vi "GlyphFactory_Init.vi"(8 "error in (no error)":errorcluster, 11 "reference in":refnum<class "GlyphFactory.lvclass"> caption="This control should only be used when\na sub class is inheriting this class") -> (0 "error out":errorcluster, 3 "reference out":refnum<class "GlyphFactory.lvclass"> caption="This indicator should only be used when\na sub class is inheriting this class")   [LabVIEW 2012, in "GlyphFactory.lvclass"]
uses:
  GlyphFactory.lvclass
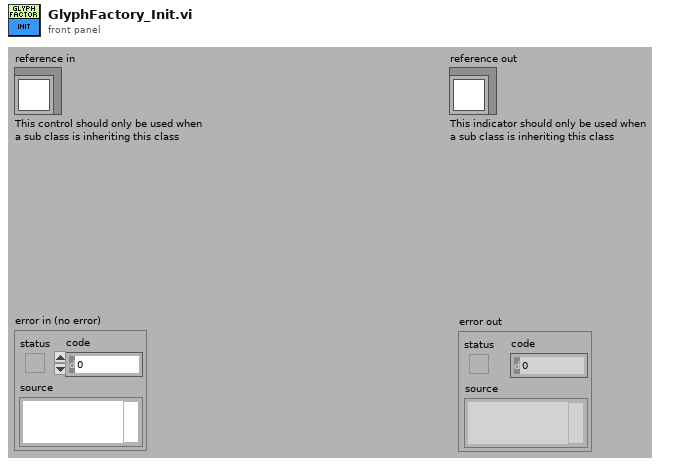
[diagram p1: front panel]
types:
  T1 = typedef "GlyphFactory.lvclass/ObjectAttributes.ctl" = cluster{"CharObjectTypes":cluster{"Char":string, "Text Color":u32, "Font":cluster{"Font Name:":string, "Size":i16, "Strikeout?":bool, "Italic?":bool, "Underline?":bool, "Outline?":bool, "Shadow?":bool, "Bold?":bool}}[], "CharObjects":refnum<class "Character.lvclass">[]}
  T2 = cluster{"Char":string, "Text Color":u32, "Font":cluster{"Font Name:":string, "Size":i16, "Strikeout?":bool, "Italic?":bool, "Underline?":bool, "Outline?":bool, "Shadow?":bool, "Bold?":bool}}[]
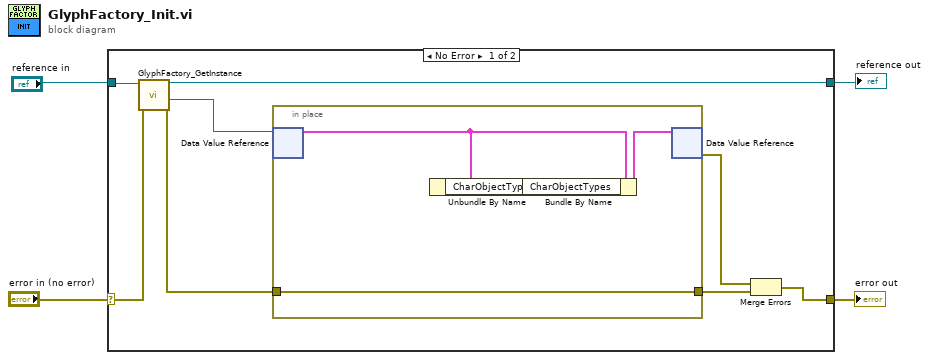
[diagram p0: block diagram]
diagram:
  n1 = case shown="No Error" "error in (no error)" {
    selector: "error in (no error)" -> [w10 w18]
    tunnel: [w11 w18] -> w3
    tunnel: "reference in" -> [w9 w17]
    tunnel: [w7 w17] -> w1
    frame No Error {
      n2 = call "GlyphFactory_GetInstance.vi"("error in (no error)"=w10, "reference in"=w9) -> ("error out"=w6:errorcluster, "DVRRefOut"=w8:refnum<data-value>, "reference out"=w7:refnum<class "GlyphFactory.lvclass">)  [unwired: 6 in, 1 out]
      n3 = in-place {
        in-place-border: w6 -> [w13]
        in-place-border: [w13] -> w5
        n4 = in-place-dvr #1(w8) -> (w15:T1)  [unwired: 1 out]
        n5 = Unbundle By Name(w15) -> ("CharObjectTypes"=w14:T2)
        n6 = Bundle By Name(cluster=w15, "CharObjectTypes"=w14) -> (w16:T1)
        n7 = in-place-dvr #1(w16) -> (w12:errorcluster)  [unwired: 1 out]
      }
      n8 = Merge Errors(w12, w5) -> (w11:errorcluster)
    }
    frame Error {
    }
  }
  "error out" <- w3
  "reference out" <- w1
